vi "ServoRange(SubVI).vi"(11 "Gray Target (-15 to -90)":i16) -> (3 "Numeric":dbl)   [LabVIEW 2017]
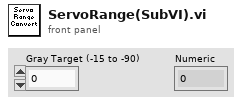
[diagram p1: front panel]
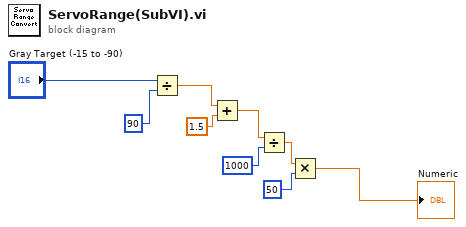
[diagram p0: block diagram]
diagram:
  n1 = Divide(x="Gray Target (-15 to -90)", y=90) -> (x/y=w2:dbl)
  n2 = Add(x=w2, y=1.5) -> (x+y=w4:dbl)
  n3 = Divide(x=w4, y=1000) -> (x/y=w6:dbl)
  n4 = Multiply(x=w6, y=50) -> (x*y=→"Numeric":dbl)
